vi "Update Water Level.vi"(8 "error in (no error)":errorcluster, 10 "Water Level":dbl, 11 "Evaporative Cooler Controller in":refnum<class "Evaporative Cooler Controller.lvclass">) -> (0 "error out":errorcluster, 3 "Evaporative Cooler Controller out":refnum<class "Evaporative Cooler Controller.lvclass">)   [LabVIEW 2025, in "Evaporative Cooler Controller.lvlib" / "Evaporative Cooler Controller.lvclass"]
doc: "Child classes should override this method to update their display or log files with the new water depth of the water basin."
uses:
  Evaporative Cooler Controller.lvclass
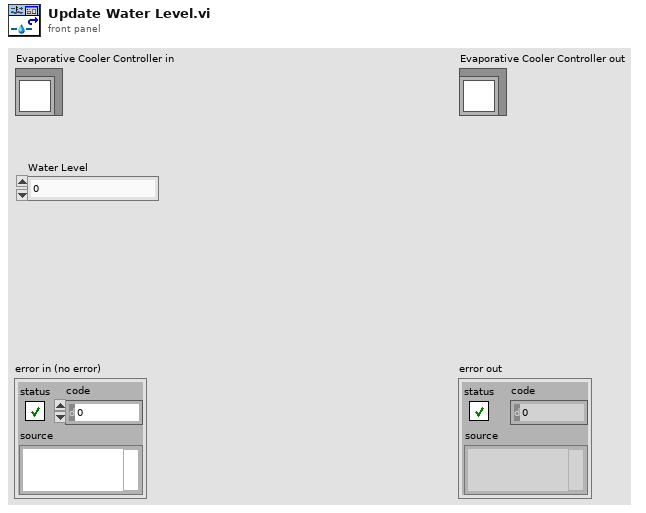
[diagram p1: front panel]
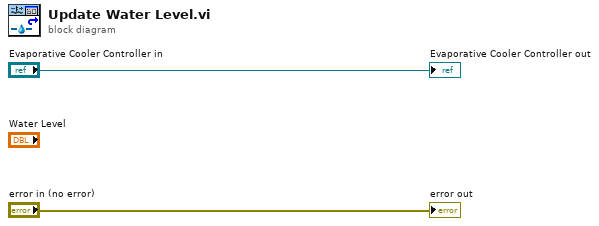
[diagram p0: block diagram]
diagram:
  "error out" <- "error in (no error)"
  "Evaporative Cooler Controller out" <- "Evaporative Cooler Controller in"
